vi "Set SLSC Switch Product Name.vi"(8 "error in (no error)":errorcluster, 10 "product name":string, 11 "SLSC Switch Custom Device Ref in":T1 format="%.0x") -> (0 "error out":errorcluster, 3 "SLSC Switch Custom Device Ref out":T1 format="%.0x")   [LabVIEW 2017, in "SLSC Switch Scripting.lvlib"]
uses:
  SLSC Switch Scripting.lvlib
  <vilib>/NI Veristand/Custom Device API/Custom Device Item Ref.ctl
  SLSC Scripting Constants.vi
  <vilib>/NI Veristand/Custom Device API/Set Item Property (String).vi
  <vilib>/NI Veristand/Custom Device API/Custom Device API.lvlib
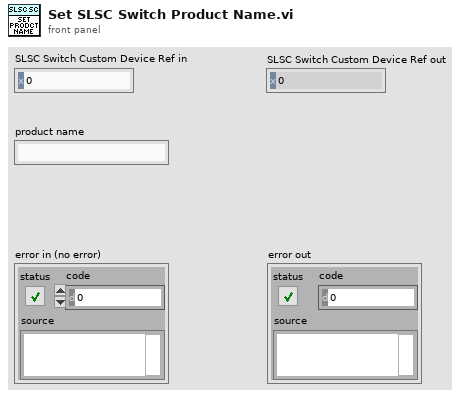
[diagram p1: front panel]
types:
  T1 = typedef "Custom Device API.lvlib/Custom Device Item Ref.ctl" = u64
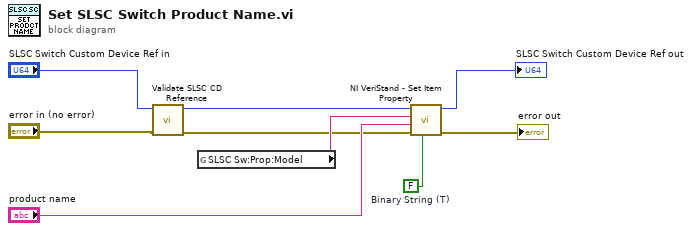
[diagram p0: block diagram]
diagram:
  w6 = FALSE  # Binary String (T)
  n1 = call "Validate SLSC CD Reference.vi"("error in (no error)"="error in (no error)", "SLSC Switch Custom Device Ref in"="SLSC Switch Custom Device Ref in") -> ("error out"=w3:errorcluster, "SLSC Switch Custom Device Ref out"=w1:T1)  [unwired: 8 in]
  n2 = global read "SLSC Scripting Constants.vi" "SLSC Sw:Prop:Model"() -> (w7:string)
  n3 = call-poly <vilib>:"NI VeriStand - Set Item Property.vi"("Binary String (T)"=w6, "error in (no error)"=w3, "Value"="product name", "Property Name"=w7, "Item Ref in"=w1) -> ("error out"=→"error out":errorcluster, "Item Ref out"=→"SLSC Switch Custom Device Ref out":T1)  [unwired: 4 in, 1 out]
